vi "NISE.Close Session.vi"(0 "SLSC Interface in":refnum<class "SLSC Interface.lvclass">, 11 "error in (no error)":errorcluster) -> (15 "error out":errorcluster)   [LabVIEW 2016, in "SLSC Interface.lvclass"]
uses:
  SLSC Interface.lvclass
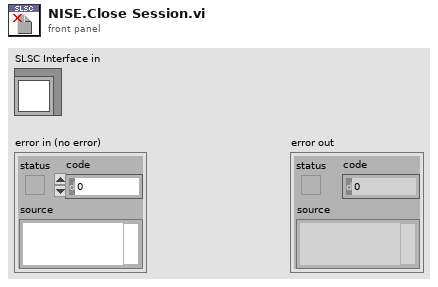
[diagram p1: front panel]
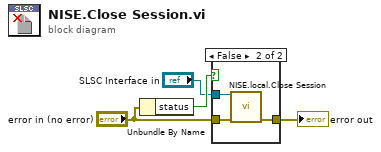
[diagram p0: block diagram]
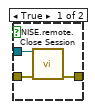
[diagram p2: hidden frame]
diagram:
  n1 = Unbundle By Name("error in (no error)") -> ("status"=w4:bool)
  n2 = case shown="False" w4 {
    tunnel: "SLSC Interface in" -> [w7 w10]
    tunnel: "error in (no error)" -> [w6 w9]
    tunnel: [w5 w8] -> w1
    frame True {
      n3 = call "NISE.remote.Close Session.vi"("SLSC Remote in"=w7, "error in (no error)"=w6) -> ("error out"=w5:errorcluster)  [unwired: 13 in]
    }
    frame False {
      n4 = call "NISE.local.Close Session.vi"("SLSC Local in"=w10, "error in (no error)"=w9) -> ("error out"=w8:errorcluster)  [unwired: 13 in]
    }
  }
  "error out" <- w1
